vi "Get Iteration.vi"(8 "error in (no error)":errorcluster, 11 "Transfer Group in":refnum<class "Transfer Group.lvclass">) -> (0 "error out":errorcluster, 2 "iteration":u64=1, 3 "Transfer Group out":refnum<class "Transfer Group.lvclass">)   [LabVIEW 2017, in "DSF Core.lvlib" / "Transfer Group.lvclass"]
uses:
  Transfer Group.lvclass
  Transfer Group.lvclass/Transfer Group.ctl
  Timing/Timing.lvclass/Timing.ctl
  Timing/Timing.lvclass
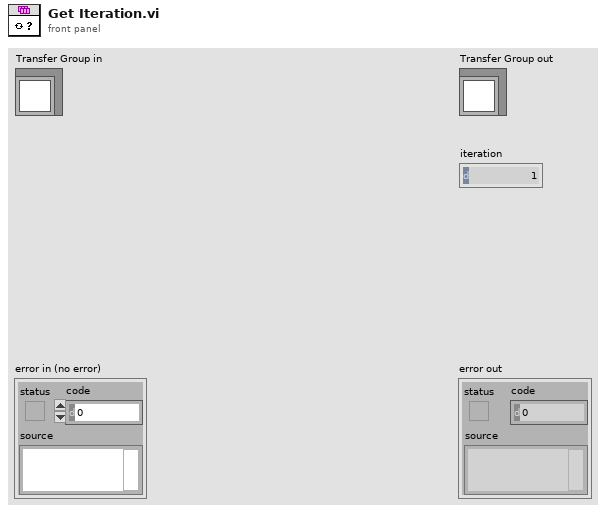
[diagram p1: front panel]
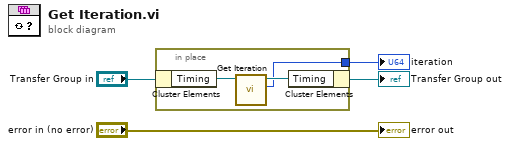
[diagram p0: block diagram]
diagram:
  n1 = in-place {
    in-place-border: [w5] -> w1
    n2 = in-place-cluster #1("Transfer Group in") -> ("Timing"=w7:refnum<class "Timing.lvclass">)
    n3 = call "Get Iteration.vi"("Timing in"=w7) -> ("Iteration"=w5:u64, "Timing out"=w6:refnum<class "Timing.lvclass">)  [unwired: 9 in]
    n4 = in-place-cluster #1("Timing"=w6) -> (→"Transfer Group out":refnum<class "Transfer Group.lvclass">)
  }
  "iteration" <- w1
  "error out" <- "error in (no error)"
